vi "find min power for turn.vi"() -> (1 "Min power":dbl)   [LabVIEW 2017]
uses:
  <vilib>/Rock Robotics/WPI/Utilities/WPI_GetSetVariantRefNum.vi
  <vilib>/Rock Robotics/WPI/RobotDrive/WPI_RobotDriveArcadeDrive_Standard(NoSaturation).vi
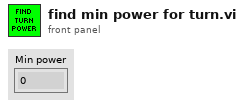
[diagram p1: front panel]
types:
  T1 = typedef "WPI_EncoderDevRef.ctl" = cluster{"DevStatus":errorcluster, "EncoderIndex":T2, "CounterIndex":T3, "DistancePerCount":dbl, "Decoding Type":T4}
  T2 = typedef "FPGA_EncoderIdx.ctl" = enum8{"Enc 0", "Enc 1", "Enc 2", "Enc 3", "Enc 4", "Enc 5", "Enc 6", "Enc 7", "Invalid"}
  T3 = typedef "FPGA_CounterCtrSystemIndex.ctl" = enum8{"Ctr 0", "Ctr 1", "Ctr 2", "Ctr 3", "Ctr 4", "Ctr 5", "Ctr 6", "Ctr 7", "Invalid"}
  T4 = typedef "WPI_EncoderType.ctl" = enum16{"1x", "2x", "4x"}
  T5 = typedef "WPI_RobotDriveDevRef.ctl" = cluster{"DevStatus":errorcluster, "Motors[]":T6[], "Square Inputs":bool, "Max Output":dbl}
  T6 = typedef "WPI_MotorControlDeviceRef.ctl" = cluster{"DeviceStatus":errorcluster, "Type":T7, "PWM":cluster{"PWM Channel":T8, "DeadBand":T9}, "CAN":cluster{"Device Number":u8, "SetOutput VI Ref":variant, "GetOutput VI Ref":variant, "Enable VI Ref":variant, "Disable VI Ref":variant, "Data":variant}, "Invert":bool, "DIO PWM":cluster{"PWM \"Enable\" Channel":T8, "DIOChannel":T10, "PWM Rate":dbl}}
  T7 = typedef "WPI_MotorControlType.ctl" = enum16{"PWM", "CAN", "DIO PWM"}
  T8 = typedef "FPGA_DIOPWMChannel.ctl" = enum8{"PWM 0", "PWM 1", "PWM 2", "PWM 3", "PWM 4", "PWM 5", "PWM 6", "PWM 7", "PWM 8", "PWM 9", "PWM MXP 0", "PWM MXP 1", "PWM MXP 2", "PWM MXP 3", "PWM MXP 4", "PWM MXP 5", "PWM MXP 6", "PWM MXP 7", "PWM MXP 8", "PWM MXP 9", "Invalid"}
  T9 = typedef "WPI_PWMDeadband.ctl" = cluster{"Name":string, "maxPositivePwm":i32, "minPositivePwm":i32, "centerPwm":i32, "maxNegativePwm":i32, "minNegativePwm":i32, "angularRange":u16}
  T10 = typedef "FPGA_DIOChannel.ctl" = enum8{"DIO 0", "DIO 1", "DIO 2", "DIO 3", "DIO 4", "DIO 5", "DIO 6", "DIO 7", "DIO 8", "DIO 9", "DIO MXP 0", "DIO MXP 1", "DIO MXP 2", "DIO MXP 3", "DIO MXP 4", "DIO MXP 5", "DIO MXP 6", "DIO MXP 7", "DIO MXP 8", "DIO MXP 9", "DIO MXP 10", "DIO MXP 11", "DIO MXP 12", "DIO MXP 13", "DIO MXP 14", "DIO MXP 15", "SPI Port CS1", "SPI Port CS2", "SPI Port CS3", "SPI Port MISO", "SPI Port MOSI", "Invalid"}
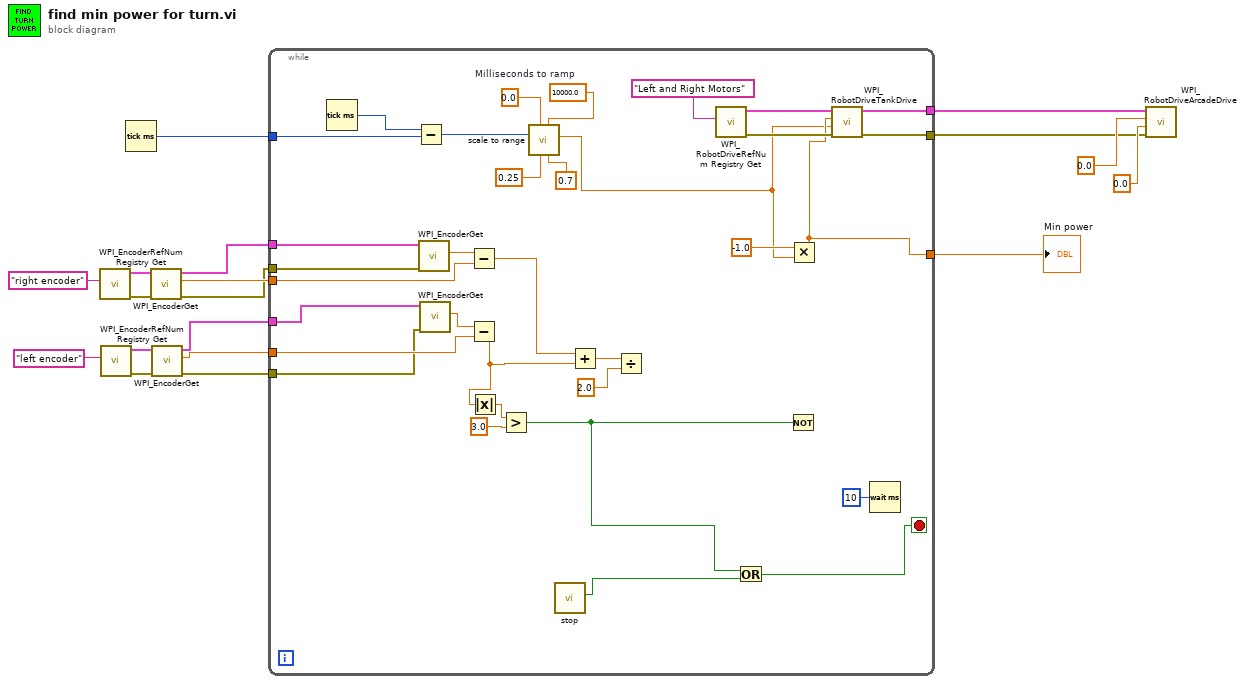
[diagram p0: block diagram]
diagram:
  n1 = call <vilib>:"WPI_EncoderRefNum Registry Get.vi"("refnum name"="right encoder") -> ("error out"=w18:errorcluster, "EncoderDevRef"=w17:T1)  [unwired: 9 in]
  n2 = call <vilib>:"WPI_EncoderRefNum Registry Get.vi"("refnum name"="left encoder") -> ("error out"=w15:errorcluster, "EncoderDevRef"=w14:T1)  [unwired: 9 in]
  n3 = Tick Count (ms)() -> (millisecond timer value=w2:u32)
  n4 = call <vilib>:"WPI_EncoderGet.vi"("error in (no error)"=w18, "EncoderDevRef"=w17) -> ("error out"=w5:errorcluster, "Distance"=w12:dbl, "EncoderDevRef"=w6:T1)  [unwired: 4 in, 3 out]
  n5 = call <vilib>:"WPI_EncoderGet.vi"("error in (no error)"=w15, "EncoderDevRef"=w14) -> ("error out"=w4:errorcluster, "Distance"=w11:dbl, "EncoderDevRef"=w3:T1)  [unwired: 4 in, 3 out]
  n6 = while {
    tunnel: w12 -> [w45]
    tunnel: w11 -> [w46]
    tunnel: [w44] -> w8
    tunnel: [w43] -> w7
    tunnel: w6 -> [w42]
    tunnel: w5 -> [w41]
    tunnel: w4 -> [w40]
    tunnel: w3 -> [w39]
    tunnel: w2 -> [w33]
    tunnel: [w23] -> w1
    stop <- w19 stop-if-true
    w30 = 10000.0  # Milliseconds to ramp
    n7 = Tick Count (ms)() -> (millisecond timer value=w32:u32)
    n8 = Subtract(x=w32, y=w33) -> (x-y=w27:u32)
    n9 = call <vilib>:"WPI_EncoderGet.vi"("error in (no error)"=w41, "EncoderDevRef"=w42) -> ("Distance"=w48:dbl)  [unwired: 4 in, 5 out]
    n10 = call <vilib>:"WPI_EncoderGet.vi"("error in (no error)"=w40, "EncoderDevRef"=w39) -> ("Distance"=w47:dbl)  [unwired: 4 in, 5 out]
    n11 = Subtract(x=w48, y=w45) -> (x-y=w36:dbl)
    n12 = Subtract(x=w47, y=w46) -> (x-y=w25:dbl)
    n13 = Absolute Value(x=w25) -> (abs(x)=w24:dbl)
    n14 = Greater?(x=w24, y=3.0) -> (0:w20:bool)
    n15 = call "scale to range.vi"("Max"=0.7 ("Min"), "High"=w30, "Min"=0.25, "Low"=0.0, "In Signal"=w27) -> ("Output signal"=w22:dbl)  [unwired: 6 in]
    n16 = call "stop.vi"() -> ("Boolean"=w21:bool)  [unwired: 11 in]
    n17 = Add(x=w36, y=w25) -> (x+y=w38:dbl)
    n18 = Divide(x=w38, y=2.0) -> ()  [unwired: 1 out]
    n19 = call <vilib>:"WPI_RobotDriveRefNum Registry Get.vi"("refnum name"="Left and Right Motors") -> ("error out"=w50:errorcluster, "RobotDriveDevRef"=w49:T5)  [unwired: 1 in, 8 out]
    n20 = Or(x=w20, y=w21) -> (x .or. y?=w19:bool)
    n21 = Not(x=w20) -> ()  [unwired: 1 out]
    n22 = Multiply(x=-1.0, y=w22) -> (x*y=w23:dbl)
    n23 = call <vilib>:"WPI_RobotDriveTankDrive.vi"("error in (no error)"=w50, "Right axis value"=w22, "Left axis value"=w23, "RobotDriveDevRef"=w49) -> ("error out"=w44:errorcluster, "RobotDriveDevRef"=w43:T5)  [unwired: 5 in, 1 out]
    n24 = Wait (ms)(milliseconds to wait=u32 10) -> ()  [unwired: 1 out]
  }
  "Min power" <- w1
  n25 = call-poly <vilib>:"WPI_RobotDriveArcadeDrive.vi"("error in (no error)"=w8, "Y axis value"=0.0 ("X axis value"), "X axis value"=0.0, "RobotDriveDevRef"=w7) -> ()  [unwired: 8 out]
